vi "Begin.vi"(11 "Image Size":T1=enum."320x240") -> (0 "error out":errorcluster)   [LabVIEW 2012]
doc: "Called before other user functions, this VI is expected to open initial I/O refnums, load in file data, and do all program initialization. Notice that the <B>error out</B> terminal is simply used for data flow. Wiring it to other structures or subVIs ensures that this VI runs first."
uses:
  <vilib>/Rock Robotics/WPI/Camera/WPI_CameraImageSize.ctl
  <vilib>/Rock Robotics/WPI/DriverStation/WPI_DriverStationRobotMode2.ctl
  <vilib>/Rock Robotics/WPI/Joystick/WPI_JoystickDeviceEnum.ctl
  <vilib>/Rock Robotics/SystemInterfaces/DIO/FPGA_DIOPWMChannel.ctl
  <vilib>/Rock Robotics/SystemInterfaces/DIO/FPGA_DIORelayChannel.ctl
  <vilib>/Rock Robotics/SystemInterfaces/DIO/FPGA_DIOChannel.ctl
  <vilib>/Rock Robotics/SystemInterfaces/Typedef/FPGA_TypedefDigitalModule.ctl
  <vilib>/Rock Robotics/WPI/Solenoid/WPI_SolenoidChannel.ctl
  <vilib>/Rock Robotics/WPI/Encoder/WPI_EncoderType.ctl
  <vilib>/Rock Robotics/SystemInterfaces/Typedef/FPGA_TypedefAnalogModule.ctl
  <vilib>/Rock Robotics/SystemInterfaces/AI/FPGA_AIChannel.ctl
  RefnameEnum.ctl
  Sally_Dashboard_2014/DBNameEnum.ctl
  <vilib>/Rock Robotics/WPI/Solenoid/WPI_SolenoidValue.ctl
  <vilib>/Rock Robotics/WPI/SafetyOutput/WPI_SafetyOutputConfigMenu.ctl
  QueueInstruction.ctl
  SubsystemEnum.ctl
  ActionEnum.ctl
  TeleopData.ctl
  <vilib>/Rock Robotics/SystemInterfaces/CounterEncoderSourceConvertion/FPGA_CounterEncoderSourceConvertionLVSourceType.ctl
  <vilib>/Rock Robotics/SystemInterfaces/DIO/FPGA_DIODigitalSourceChannel.ctl
  <vilib>/Rock Robotics/SystemInterfaces/AnalogTrigger/FPGA_AnalogTriggerIndex.ctl
  <vilib>/Rock Robotics/SystemInterfaces/AnalogTrigger/FPGA_AnalogTriggerOutType.ctl
  Robot Global Data.vi
  <vilib>/Rock Robotics/WPI/RobotDrive/WPI_RobotDriveOpen2MotorWithTalon.vi
  <vilib>/Rock Robotics/WPI/MotorControl/WPI_MotorControlOpen Talon.vi
  <vilib>/Rock Robotics/WPI/Counter/WPI_CounterDigitalInputToDigitalSource.vi
  <vilib>/Rock Robotics/WPI/Solenoid/WPI_SolenoidOpenSingle.vi
  <vilib>/Rock Robotics/WPI/Solenoid/WPI_SolenoidSetEnum.vi
  <vilib>/Rock Robotics/WPI/MotorControl/WPI_MotorControlOpen Jaguar.vi
  <vilib>/Rock Robotics/WPI/Compressor/WPI_CompressorGetSetRefNum.vi
  <vilib>/Rock Robotics/WPI/Counter/WPI_CounterOpen UpDown Mode.vi
  <vilib>/Rock Robotics/WPI/Camera/WPI_CameraWhite Balance Values.ctl
  <vilib>/Rock Robotics/WPI/Camera/WPI_CameraExposure Values.ctl
  <vilib>/Rock Robotics/WPI/Camera/WPI_CameraFrameRate.ctl
  <vilib>/Rock Robotics/SystemInterfaces/AI/FPGA_AIGyroChannel.ctl
  <vilib>/Rock Robotics/SystemInterfaces/Typedef/FPGA_TypedefAnalogModuleForGyro.ctl
panel:
  in  "LowerLimit (v)":dbl=-1.0
  in  "UpperLimit (v)":dbl=1.0
  out "error out 2":errorcluster
  in  "Version String":string="TruongFramework 1.5.2"
  # "DON'T FORGET TO MAKE THIS DEFAULT"
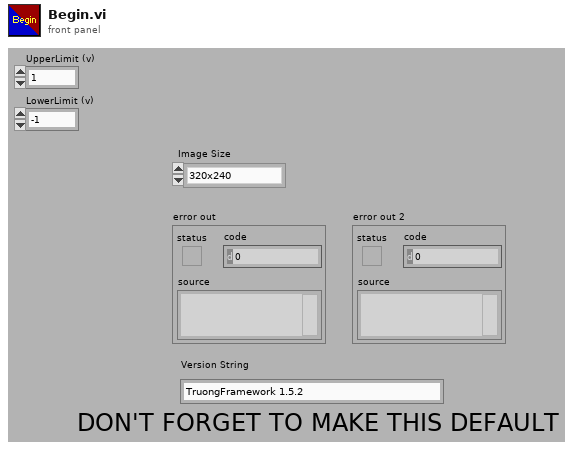
[diagram p1: front panel]
types:
  T1 = typedef "WPI_CameraImageSize.ctl" = enum16{"640x480", "320x240", "160x120"}
  T2 = typedef "TeleopData.ctl" = cluster{"cTankDriveLeft":dbl, "cTankDriveRight":dbl, "cHalfSpeed":bool, "cClimbWeight":bool, "cClimbStart":bool, "cRpmControl":dbl, "cAngleControl":dbl, "cQuickShoot":bool, "cLauncherWheel":bool, "cFirePneumatic":bool, "cPresetLow":bool, "cPresetHigh":bool, "cPresetClimbLow":bool, "cPresetClimbHigh":bool, "cLauncherAngle":bool, "cResetAngleEncoder":bool}
  T3 = typedef "QueueInstruction.ctl" = cluster{"Data":variant, "Subsystem":T4, "Action":T5}
  T4 = typedef "SubsystemEnum.ctl" = enum16{"TankDrive", "FirePneumatic", "Climber", "ClimbWeight", "ShooterAngle"}
  T5 = typedef "ActionEnum.ctl" = enum16{"Init", "SetValue"}
  T6 = typedef "WPI_SafetyOutputConfigMenu.ctl" = enum16{"Enable", "Disable"}
  T7 = typedef "WPI_SolenoidValue.ctl" = enum16{"Off", "On", "Forward", "Reverse"}
  T8 = typedef "RefnameEnum.ctl" = enum16{"FireLauncher", "Climber", "Shield", "TankDrive", "DriveEncoderL", "DriveEncoderR", "LauncherMotorRPM", "LauncherEncoderAnalog", "LauncherEncoderRPM", "ShooterLS", "DriveAlignLSLeft", "DriveAlignLSRight", "ClimbingLS", "LauncherEncoderAngle", "LauncherMotorAngle", "Gamepad1", "Gamepad2", "Compressor", "ClimbWeightSol3", "ClimbWeightSol4"}
  T9 = typedef "WPI_SolenoidChannel.ctl" = enum8{"Solenoid 1", "Solenoid 2", "Solenoid 3", "Solenoid 4", "Solenoid 5", "Solenoid 6", "Solenoid 7", "Solenoid 8", "Invalid"}
  T10 = typedef "FPGA_DIOChannel.ctl" = enum8{"DIO 1", "DIO 2", "DIO 3", "DIO 4", "DIO 5", "DIO 6", "DIO 7", "DIO 8", "DIO 9", "DIO 10", "DIO 11", "DIO 12", "DIO 13", "DIO 14", "Invalid"}
  T11 = typedef "FPGA_TypedefDigitalModule.ctl" = enum16{"Digital Module 1", "Digital Module 2"}
  T12 = typedef "DBNameEnum.ctl" = enum16{"AutoInstructions", "DriveLoopTime", "DriveAlignLSLeft", "DriveAlignLSRight", "Use2DriveAlign", "ClimbLS", "LauncherAngleMatches", "FrameworkVersion", "sLauncherAngle", "LauncherTargetAngle", "sLauncherRPM", "LauncherTargetRPM", "sDriveDistance", "LauncherMotorValue", "PullbackTol", "FireTol", "LauncherRPMTol", "LauncherAngleTol", "InitialWait", "WaitBetweenLaunch", "AnglePresets", "RPMPresets", "UseAngleEncoder", "UseLauncherEncoder", "UseLauncherPID", "QSWaitBeforeFire", "QSWaitBeforeRetract", "AngleForwardValue", "AngleBackwardValue", "UseClusterArray", "BackupAuto", "ReverseDriveIndicate", "HalfSpeedFactor"}
  T13 = typedef "FPGA_AIChannel.ctl" = enum8{"AI 1", "AI 2", "AI 3", "AI 4", "AI 5", "AI 6", "AI 7", "AI 8", "Invalid"}
  T14 = typedef "FPGA_TypedefAnalogModule.ctl" = enum16{"Analog Module 1", "Analog Module 2"}
  T15 = typedef "WPI_EncoderType.ctl" = enum16{"1x", "2x", "4x"}
  T16 = typedef "FPGA_DIORelayChannel.ctl" = enum8{"Relay 1", "Relay 2", "Relay 3", "Relay 4", "Relay 5", "Relay 6", "Relay 7", "Relay 8", "Invalid"}
  T17 = typedef "FPGA_DIOPWMChannel.ctl" = enum8{"PWM 1", "PWM 2", "PWM 3", "PWM 4", "PWM 5", "PWM 6", "PWM 7", "PWM 8", "PWM 9", "PWM 10", "Invalid"}
  T18 = typedef "WPI_JoystickDeviceEnum.ctl" = enum16{"USB 1", "USB 2", "USB 3", "USB 4", "Kinect 1", "Kinect 2"}
  T19 = typedef "WPI_DriverStationRobotMode2.ctl" = enum16{"Autonomous Disabled", "Autonomous Enabled", "Teleop Disabled", "Teleop Enabled", "Timeout", "Finish", "Test Disabled", "Test Enabled"}
  T20 = enum16{"Rising Edge", "Falling Edge", "Raising & Falling Edge", "Disabled"}
  T21 = typedef "WPI_DigitalInputDevRef.ctl" = cluster{"DevStatus":errorcluster, "DIO Channel":T10, "Digital Module":T11}
  T22 = typedef "FPGA_CounterEncoderSourceConvertionLVSourceType.ctl" = cluster{"DevStatus":errorcluster, "AnalogTriggerMode?":bool, "DigitalMode":cluster{"Digital Module":T11, "DIO Channel":T23}, "AnalogTriggerMode":cluster{"AnalogTriggerIndex":T24, "OutputType":T25}}
  T23 = typedef "FPGA_DIODigitalSourceChannel.ctl" = enum8{"DIO 1", "DIO 2", "DIO 3", "DIO 4", "DIO 5", "DIO 6", "DIO 7", "DIO 8", "DIO 9", "DIO 10", "DIO 11", "DIO 12", "DIO 13", "DIO 14", "Disabled"}
  T24 = typedef "FPGA_AnalogTriggerIndex.ctl" = enum8{"Trig 0", "Trig 1", "Trig 2", "Trig 3", "Trig 4", "Trig 5", "Trig 6", "Trig 7", "Invalid"}
  T25 = typedef "FPGA_AnalogTriggerOutType.ctl" = enum16{"InWindow", "TriggerState", "Rising", "Falling"}
  T26 = typedef "WPI_EncoderDevRef.ctl" = cluster{"DevStatus":errorcluster, "EncoderIndex":T27, "CounterIndex":T28, "DistancePerCount":dbl, "Decoding Type":T15}
  T27 = typedef "FPGA_EncoderIdx.ctl" = enum8{"Enc 0", "Enc 1", "Enc 2", "Enc 3", "Invalid"}
  T28 = typedef "FPGA_CounterCtrSystemIndex.ctl" = enum8{"Ctr 0", "Ctr 1", "Ctr 2", "Ctr 3", "Ctr 4", "Ctr 5", "Ctr 6", "Ctr 7", "Invalid"}
  T29 = typedef "WPI_CounterDevRef.ctl" = cluster{"DevStatus":errorcluster, "CntIndex":T28}
  T30 = typedef "FPGA_AIGyroChannel.ctl" = enum8{"AI 1", "AI 2", "Invalid"}
  T31 = typedef "FPGA_TypedefAnalogModuleForGyro.ctl" = enum16{"Analog Module 1"}
  T32 = typedef "WPI_GyroDevRef.ctl" = cluster{"DevStatus":errorcluster, "Analog Module":T14, "Analog Channel":T13, "Offset":dbl, "Gain (VoltsPerDegree/Second)":dbl}
  T33 = typedef "WPI_MotorControlDeviceRef.ctl" = cluster{"DeviceStatus":errorcluster, "Type":enum16{"PWM", "CAN"}, "PWM":cluster{"Digital Module":T11, "PWM Channel":T17, "DeadBand":T34}, "CAN":cluster{"Device Number":u8, "Control Mode":T35, "Semaphore":T36, "Max Vout":dbl}, "Invert":bool, "TransformRef":T37, "InvTransformRef":T37}
  T34 = typedef "WPI_PWMDeadband.ctl" = cluster{"Name":string, "maxPositivePwm":i32, "minPositivePwm":i32, "centerPwm":i32, "maxNegativePwm":i32, "minNegativePwm":i32, "angularRange":u16}
  T35 = typedef "WPI_CANJaguar_ControlMode.ctl" = enum8{"Percent VBus", "Current", "Speed", "Position", "Voltage"}
  T36 = typedef "Semaphore RefNum" = refnum<k1>
  T37 = typedef "WPI_PWMTransform_ConPane.ctl" = refnum<vi>
  T38 = typedef "WPI_RelayDevRef.ctl" = cluster{"DevStatus":errorcluster, "Relay Channel":T16, "Digital Module":T11, "Relay Direction":T39}
  T39 = typedef "WPI_RelayDirection.ctl" = enum16{"Both directions", "Forward only", "Reverse only"}
  T40 = typedef "WPI_SolenoidDevRef.ctl" = cluster{"DevStatus":errorcluster, "Solenoid Module":T41, "Forward Solenoid Channel":T9, "Reverse Solenoid Channel":T9}
  T41 = typedef "FPGA_TypedefSolenoidModule.ctl" = enum16{"Solenoid Module 1", "Solenoid Module 2"}
  T42 = typedef "WPI_CompressorDevRef.ctl" = cluster{"DevStatus":errorcluster, "DigitalInputDevRef":T21, "RelayDevRef":T38}
  T43 = typedef "WPI_RobotDriveDevRef.ctl" = cluster{"DevStatus":errorcluster, "Motors[]":T33[], "Square Inputs":bool, "Max Output":dbl, "Isochronous":bool}
  T44 = typedef "WPI_CameraFrameRate.ctl" = u32
  T45 = typedef "WPI_CameraExposure Values.ctl" = enum16{"Auto", "Flicker-free 50 Hz", "Flicker-free 60 Hz", "Hold current"}
  T46 = typedef "WPI_CameraWhite Balance Values.ctl" = enum16{"Auto", "Fixed indoor", "Fixed outdoor 1", "Fixed outdoor 2", "Fixed fluorescent 1", "Fixed fluorescent 2", "Hold current"}
  T47 = typedef "WPI_CameraDevRef.ctl" = cluster{"Camera Address":string, "CameraStatus":errorcluster, "Acquire Image Notifier":refnum<notifier>}
  T48 = typedef "WPI_JoystickDevRef.ctl" = cluster{"Device":T18}
  T49 = typedef "WPI_AnalogChannelDevRef.ctl" = cluster{"DevStatus":errorcluster, "Analog Module":T14, "Analog Channel":T13}
  T50 = typedef "FPGA_AnalogTriggerDevRef.ctl" = cluster{"DevStatus":errorcluster, "AnalogTriggerIndex":T24}
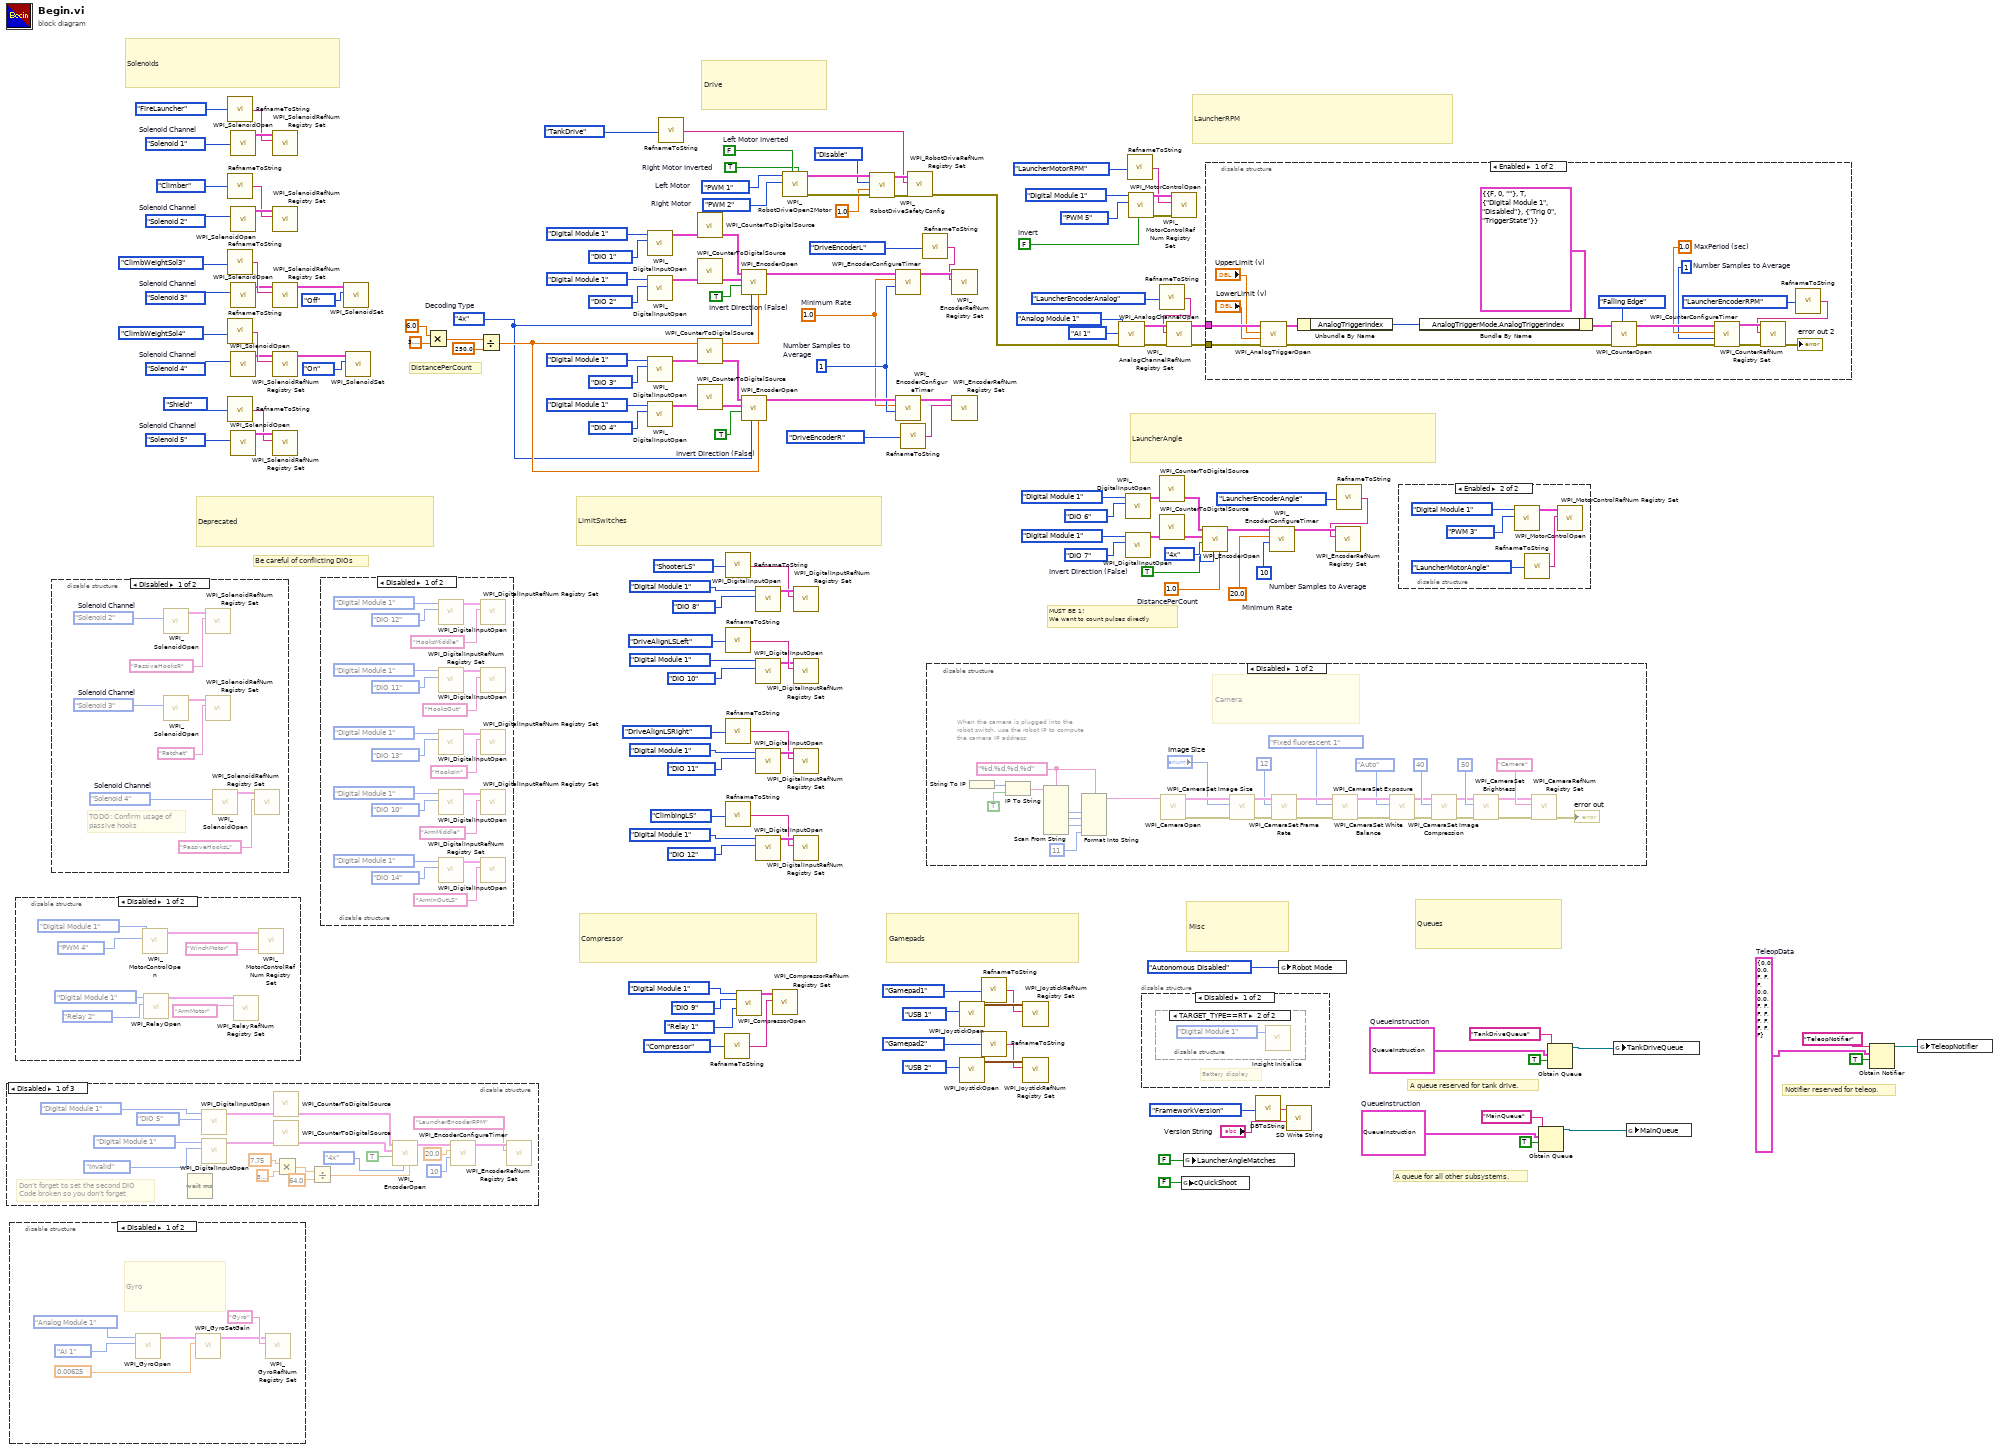
[diagram p0: block diagram]
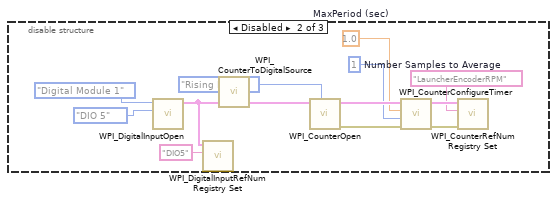
[diagram p8: hidden frame]
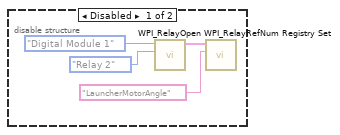
[diagram p12: hidden frame]
diagram:
  w4 = T2 {"cTankDriveLeft"=0.0, "cTankDriveRight"=0.0, "cHalfSpeed"=FALSE, "cClimbWeight"=FALSE, "cClimbStart"=FALSE, "cRpmControl"=0.0, "cAngleControl"=0.0, "cQuickShoot"=FALSE, "cLauncherWheel"=FALSE, "cFirePneumatic"=FALSE, "cPresetLow"=FALSE, "cPresetHigh"=FALSE, "cPresetClimbLow"=FALSE, "cPresetClimbHigh"=FALSE, "cLauncherAngle"=FALSE, "cResetAngleEncoder"=FALSE}  # TeleopData
  w9 = T3 {"Data"=variant, "Subsystem"=enum."TankDrive", "Action"=enum."Init"}  # QueueInstruction
  w10 = T3 {"Data"=variant, "Subsystem"=enum."TankDrive", "Action"=enum."Init"}  # QueueInstruction
  w24 = WPI_SolenoidChannel."Solenoid 4"  # Solenoid Channel
  w28 = WPI_SolenoidChannel."Solenoid 3"  # Solenoid Channel
  w84 = 1.0  # DistancePerCount
  w87 = TRUE  # Invert Direction (False)
  w88 = TRUE  # Invert Direction (False)
  w92 = WPI_SolenoidChannel."Solenoid 5"  # Solenoid Channel
  w94 = WPI_SolenoidChannel."Solenoid 2"  # Solenoid Channel
  w99 = TRUE  # Invert Direction (False)
  w101 = u8 10  # Number Samples to Average
  w102 = 20.0  # Minimum Rate
  w114 = WPI_SolenoidChannel."Solenoid 1"  # Solenoid Channel
  w89 = WPI_EncoderType."4x"  # Decoding Type
  w86 = u8 1  # Number Samples to Average
  w85 = 1.0  # Minimum Rate
  w143 = FALSE  # Invert
  w147 = FPGA_DIOPWMChannel."PWM 2"  # Right Motor
  w148 = FPGA_DIOPWMChannel."PWM 1"  # Left Motor
  w149 = TRUE  # Right Motor Inverted
  w150 = FALSE  # Left Motor Inverted
  # "Notifier reserved for teleop."
  # "A queue reserved for tank drive."
  # "A queue for all other subsystems."
  # "Queues"
  # "Be careful of conflicting DIOs"
  # "DistancePerCount"
  # "Deprecated"
  # "LimitSwitches"
  # "Compressor"
  # "Solenoids"
  # "LauncherAngle"
  # "LauncherRPM"
  # "Misc"
  # "Gamepads"
  # "Drive"
  # "MUST BE 1!\nWe want to count pulses directly"
  n1 = disable-structure shown="Disabled" {
    frame Disabled {
      # "Don't forget to set the second DIO\nCode broken so you don't forget"
      n2 = Wait (ms)() -> ()  [unwired: 1 in, 1 out]
      n3 = call <vilib>:"WPI_DigitalInputOpen.vi"("DIO Channel"=FPGA_DIOChannel."DIO 5", "Digital Module (Module 1)"=FPGA_TypedefDigitalModule."Digital Module 1") -> ("DigitalInputDevRef"=w173:T21)  [unwired: 1 in, 8 out]
      n4 = call <vilib>:"WPI_DigitalInputOpen.vi"("DIO Channel"=FPGA_DIOChannel."Invalid", "Digital Module (Module 1)"=FPGA_TypedefDigitalModule."Digital Module 1") -> ("DigitalInputDevRef"=w174:T21)  [unwired: 1 in, 8 out]
      n5 = call-poly <vilib>:"WPI_CounterToDigitalSource.vi"("DigitalInputDevRef"=w173) -> ("Digital Source"=w172:T22)  [unwired: 6 out]
      n6 = call-poly <vilib>:"WPI_CounterToDigitalSource.vi"("DigitalInputDevRef"=w174) -> ("Digital Source"=w175:T22)  [unwired: 6 out]
      n7 = Multiply(x=7.75, y=3.141592653589793) -> (x*y=w157:dbl)
      n8 = Divide(x=w157, y=64.0) -> (x/y=w160:dbl)
      n9 = call <vilib>:"WPI_EncoderOpen.vi"("DistancePerCount"=w160, "Decoding Type"=WPI_EncoderType."4x", "Invert Direction (False)"=TRUE, "BSource"=w175, "ASource"=w172) -> ("EncoderDevRef"=w169:T26)  [unwired: 3 in, 3 out]
      n10 = call <vilib>:"WPI_EncoderConfigureTimer.vi"("Number Samples to Average"=u8 10, "Minimum Rate"=20.0, "EncoderDevRef"=w169) -> ("EncoderDevRef"=w166:T26)  [unwired: 1 in, 7 out]
      n11 = call <vilib>:"WPI_EncoderRefNum Registry Set.vi"("refnum name"="LauncherEncoderRPM", "EncoderDevRef"=w166) -> ()  [unwired: 8 in, 2 out]
    }
    frame Disabled {
      w186 = u8 1  # Number Samples to Average
      w187 = 1.0  # MaxPeriod (sec)
      n12 = call <vilib>:"WPI_DigitalInputOpen.vi"("DIO Channel"=FPGA_DIOChannel."DIO 5", "Digital Module (Module 1)"=FPGA_TypedefDigitalModule."Digital Module 1") -> ("DigitalInputDevRef"=w177:T21)  [unwired: 8 in, 1 out]
      n13 = call <vilib>:"WPI_DigitalInputRefNum Registry Set.vi"("refnum name"="DIO5", "DigitalInputDevRef"=w177) -> ()  [unwired: 8 in, 2 out]
      n14 = call-poly <vilib>:"WPI_CounterToDigitalSource.vi"("DigitalInputDevRef"=w177) -> ("Digital Source"=w180:T22)  [unwired: 6 out]
      n15 = call-poly <vilib>:"WPI_CounterOpen.vi"("UpEdge"=T20."Rising Edge", "Up Source"=w180) -> ("error out"=w182:errorcluster, "CounterDevRef"=w188:T29)  [unwired: 8 in]
      n16 = call <vilib>:"WPI_CounterConfigureTimer.vi"("error in (no error)"=w182, "Number Samples to Average"=w186, "MaxPeriod (sec)"=w187, "CounterDevRef in"=w188) -> ("error out"=w181:errorcluster, "CounterDevRef out"=w185:T29)  [unwired: 6 in]
      n17 = call <vilib>:"WPI_CounterRefNum Registry Set.vi"("error in (no error)"=w181, "refnum name"="LauncherEncoderRPM", "CounterDevRef"=w185) -> ()  [unwired: 7 in, 2 out]
    }
    frame Enabled {
      # "LauncherRPM Deprecated"
    }
  }
  n18 = disable-structure shown="Disabled" {
    frame Disabled {
      # "Gyro"
      n19 = call <vilib>:"WPI_GyroOpen.vi"("Analog Channel"=FPGA_AIGyroChannel."AI 1", "Analog Module (Module 1)"=FPGA_TypedefAnalogModuleForGyro."Analog Module 1") -> ("GyroDevRef"=w191:T32)  [unwired: 7 in, 2 out]
      n20 = call <vilib>:"WPI_GyroSetGain.vi"("Gain (VoltsPerDegree/Second)"=0.00625, "GyroDevRef"=w191) -> ("GyroDevRef"=w190:T32)  [unwired: 8 in, 1 out]
      n21 = call <vilib>:"WPI_GyroRefNum Registry Set.vi"("refnum name"="Gyro", "GyroDevRef"=w190) -> ()  [unwired: 8 in, 2 out]
    }
    frame Enabled {
    }
  }
  n22 = disable-structure shown="Disabled" {
    frame Disabled {
      n23 = call-poly <vilib>:"WPI_MotorControlOpen.vi"("PWM Channel"=FPGA_DIOPWMChannel."PWM 4", "Digital Module (Module 1)"=FPGA_TypedefDigitalModule."Digital Module 1") -> ("MotorControlDeviceRef"=w200:T33)  [unwired: 8 in, 1 out]
      n24 = call <vilib>:"WPI_RelayOpen.vi"("Relay Channel"=FPGA_DIORelayChannel."Relay 2", "Digital Module (Module 1)"=FPGA_TypedefDigitalModule."Digital Module 1") -> ("RelayDevRef"=w196:T38)  [unwired: 8 in, 1 out]
      n25 = call <vilib>:"WPI_RelayRefNum Registry Set.vi"("refnum name"="ArmMotor", "RelayDevRef"=w196) -> ()  [unwired: 8 in, 2 out]
      n26 = call <vilib>:"WPI_MotorControlRefNum Registry Set.vi"("refnum name"="WinchMotor", "MotorControlDevRef"=w200) -> ()  [unwired: 8 in, 2 out]
    }
    frame Enabled {
    }
  }
  n27 = disable-structure shown="Disabled" {
    frame Disabled {
      w205 = WPI_SolenoidChannel."Solenoid 2"  # Solenoid Channel
      w208 = WPI_SolenoidChannel."Solenoid 4"  # Solenoid Channel
      w211 = WPI_SolenoidChannel."Solenoid 3"  # Solenoid Channel
      # "TODO: Confirm usage of\npassive hooks"
      n28 = call-poly <vilib>:"WPI_SolenoidOpen.vi"("Solenoid Channel"=w205) -> ("SolenoidDevRef"=w204:T40)  [unwired: 2 in, 8 out]
      n29 = call-poly <vilib>:"WPI_SolenoidOpen.vi"("Solenoid Channel"=w211) -> ("SolenoidDevRef"=w210:T40)  [unwired: 2 in, 8 out]
      n30 = call <vilib>:"WPI_SolenoidRefNum Registry Set.vi"("refnum name"="PassiveHooksR", "SolenoidDevRef"=w204) -> ()  [unwired: 8 in, 2 out]
      n31 = call <vilib>:"WPI_SolenoidRefNum Registry Set.vi"("refnum name"="Ratchet", "SolenoidDevRef"=w210) -> ()  [unwired: 8 in, 2 out]
      n32 = call-poly <vilib>:"WPI_SolenoidOpen.vi"("Solenoid Channel"=w208) -> ("SolenoidDevRef"=w207:T40)  [unwired: 2 in, 8 out]
      n33 = call <vilib>:"WPI_SolenoidRefNum Registry Set.vi"("refnum name"="PassiveHooksL", "SolenoidDevRef"=w207) -> ()  [unwired: 8 in, 2 out]
    }
    frame Enabled {
    }
  }
  n34 = call "RefnameToString.vi"("Enum"=RefnameEnum."FireLauncher") -> ("Refname"=w67:string)
  n35 = call "RefnameToString.vi"("Enum"=RefnameEnum."Climber") -> ("Refname"=w65:string)
  n36 = call "RefnameToString.vi"("Enum"=RefnameEnum."ClimbWeightSol3") -> ("Refname"=w31:string)
  n37 = call "RefnameToString.vi"("Enum"=RefnameEnum."ClimbWeightSol4") -> ("Refname"=w27:string)
  n38 = call "RefnameToString.vi"("Enum"=RefnameEnum."Shield") -> ("Refname"=w63:string)
  n39 = call-poly <vilib>:"WPI_SolenoidOpen.vi"("Solenoid Channel"=w114) -> ("SolenoidDevRef"=w113:T40)  [unwired: 2 in, 8 out]
  n40 = call-poly <vilib>:"WPI_SolenoidOpen.vi"("Solenoid Channel"=w94) -> ("SolenoidDevRef"=w93:T40)  [unwired: 2 in, 8 out]
  n41 = call-poly <vilib>:"WPI_SolenoidOpen.vi"("Solenoid Channel"=w28) -> ("SolenoidDevRef"=w29:T40)  [unwired: 2 in, 8 out]
  n42 = call-poly <vilib>:"WPI_SolenoidOpen.vi"("Solenoid Channel"=w24) -> ("SolenoidDevRef"=w25:T40)  [unwired: 2 in, 8 out]
  n43 = call-poly <vilib>:"WPI_SolenoidOpen.vi"("Solenoid Channel"=w92) -> ("SolenoidDevRef"=w91:T40)  [unwired: 2 in, 8 out]
  n44 = call <vilib>:"WPI_SolenoidRefNum Registry Set.vi"("refnum name"=w67, "SolenoidDevRef"=w113) -> ()  [unwired: 8 in, 2 out]
  n45 = call <vilib>:"WPI_SolenoidRefNum Registry Set.vi"("refnum name"=w65, "SolenoidDevRef"=w93) -> ()  [unwired: 8 in, 2 out]
  n46 = call <vilib>:"WPI_SolenoidRefNum Registry Set.vi"("refnum name"=w31, "SolenoidDevRef"=w29) -> ("SolenoidDevRef"=w23:T40)  [unwired: 8 in, 1 out]
  n47 = call <vilib>:"WPI_SolenoidRefNum Registry Set.vi"("refnum name"=w27, "SolenoidDevRef"=w25) -> ("SolenoidDevRef"=w22:T40)  [unwired: 8 in, 1 out]
  n48 = call <vilib>:"WPI_SolenoidRefNum Registry Set.vi"("refnum name"=w63, "SolenoidDevRef"=w91) -> ()  [unwired: 8 in, 2 out]
  n49 = disable-structure shown="Disabled" {
    frame Disabled {
      n50 = call <vilib>:"WPI_DigitalInputOpen.vi"("DIO Channel"=FPGA_DIOChannel."DIO 12", "Digital Module (Module 1)"=FPGA_TypedefDigitalModule."Digital Module 1") -> ("DigitalInputDevRef"=w215:T21)  [unwired: 8 in, 1 out]
      n51 = call <vilib>:"WPI_DigitalInputOpen.vi"("DIO Channel"=FPGA_DIOChannel."DIO 11", "Digital Module (Module 1)"=FPGA_TypedefDigitalModule."Digital Module 1") -> ("DigitalInputDevRef"=w219:T21)  [unwired: 8 in, 1 out]
      n52 = call <vilib>:"WPI_DigitalInputOpen.vi"("DIO Channel"=FPGA_DIOChannel."DIO 13", "Digital Module (Module 1)"=FPGA_TypedefDigitalModule."Digital Module 1") -> ("DigitalInputDevRef"=w223:T21)  [unwired: 8 in, 1 out]
      n53 = call <vilib>:"WPI_DigitalInputOpen.vi"("DIO Channel"=FPGA_DIOChannel."DIO 10", "Digital Module (Module 1)"=FPGA_TypedefDigitalModule."Digital Module 1") -> ("DigitalInputDevRef"=w227:T21)  [unwired: 8 in, 1 out]
      n54 = call <vilib>:"WPI_DigitalInputOpen.vi"("DIO Channel"=FPGA_DIOChannel."DIO 14", "Digital Module (Module 1)"=FPGA_TypedefDigitalModule."Digital Module 1") -> ("DigitalInputDevRef"=w231:T21)  [unwired: 8 in, 1 out]
      n55 = call <vilib>:"WPI_DigitalInputRefNum Registry Set.vi"("refnum name"="HooksMiddle", "DigitalInputDevRef"=w215) -> ()  [unwired: 8 in, 2 out]
      n56 = call <vilib>:"WPI_DigitalInputRefNum Registry Set.vi"("refnum name"="HooksOut", "DigitalInputDevRef"=w219) -> ()  [unwired: 8 in, 2 out]
      n57 = call <vilib>:"WPI_DigitalInputRefNum Registry Set.vi"("refnum name"="HooksIn", "DigitalInputDevRef"=w223) -> ()  [unwired: 8 in, 2 out]
      n58 = call <vilib>:"WPI_DigitalInputRefNum Registry Set.vi"("refnum name"="ArmMiddle", "DigitalInputDevRef"=w227) -> ()  [unwired: 8 in, 2 out]
      n59 = call <vilib>:"WPI_DigitalInputRefNum Registry Set.vi"("refnum name"="ArmInOutLS", "DigitalInputDevRef"=w231) -> ()  [unwired: 8 in, 2 out]
    }
    frame Enabled {
    }
  }
  n60 = call-poly <vilib>:"WPI_SolenoidSet.vi"("Value"=WPI_SolenoidValue."Off", "SolenoidDevRef"=w23) -> ()  [unwired: 8 in, 2 out]
  n61 = call-poly <vilib>:"WPI_SolenoidSet.vi"("Value"=WPI_SolenoidValue."On", "SolenoidDevRef"=w22) -> ()  [unwired: 8 in, 2 out]
  n62 = Multiply(x=6.0, y=3.141592653589793) -> (x*y=w96:dbl)
  n63 = Divide(x=w96, y=250.0) -> (x/y=w90:dbl)
  n64 = call <vilib>:"WPI_DigitalInputOpen.vi"("DIO Channel"=FPGA_DIOChannel."DIO 1", "Digital Module (Module 1)"=FPGA_TypedefDigitalModule."Digital Module 1") -> ("DigitalInputDevRef"=w135:T21)  [unwired: 1 in, 8 out]
  n65 = call <vilib>:"WPI_DigitalInputOpen.vi"("DIO Channel"=FPGA_DIOChannel."DIO 2", "Digital Module (Module 1)"=FPGA_TypedefDigitalModule."Digital Module 1") -> ("DigitalInputDevRef"=w136:T21)  [unwired: 1 in, 8 out]
  n66 = call <vilib>:"WPI_DigitalInputOpen.vi"("DIO Channel"=FPGA_DIOChannel."DIO 3", "Digital Module (Module 1)"=FPGA_TypedefDigitalModule."Digital Module 1") -> ("DigitalInputDevRef"=w122:T21)  [unwired: 1 in, 8 out]
  n67 = call <vilib>:"WPI_DigitalInputOpen.vi"("DIO Channel"=FPGA_DIOChannel."DIO 4", "Digital Module (Module 1)"=FPGA_TypedefDigitalModule."Digital Module 1") -> ("DigitalInputDevRef"=w123:T21)  [unwired: 1 in, 8 out]
  n68 = call "RefnameToString.vi"("Enum"=RefnameEnum."TankDrive") -> ("Refname"=w15:string)
  n69 = call-poly <vilib>:"WPI_CounterToDigitalSource.vi"("DigitalInputDevRef"=w135) -> ("Digital Source"=w134:T22)  [unwired: 6 out]
  n70 = call-poly <vilib>:"WPI_CounterToDigitalSource.vi"("DigitalInputDevRef"=w136) -> ("Digital Source"=w137:T22)  [unwired: 6 out]
  n71 = call-poly <vilib>:"WPI_CounterToDigitalSource.vi"("DigitalInputDevRef"=w122) -> ("Digital Source"=w121:T22)  [unwired: 6 out]
  n72 = call-poly <vilib>:"WPI_CounterToDigitalSource.vi"("DigitalInputDevRef"=w123) -> ("Digital Source"=w124:T22)  [unwired: 6 out]
  n73 = call "RefnameToString.vi"("Enum"=RefnameEnum."Compressor") -> ("Refname"=w44:string)
  n74 = call "RefnameToString.vi"("Enum"=RefnameEnum."ShooterLS") -> ("Refname"=w50:string)
  n75 = call "RefnameToString.vi"("Enum"=RefnameEnum."DriveAlignLSLeft") -> ("Refname"=w37:string)
  n76 = call "RefnameToString.vi"("Enum"=RefnameEnum."DriveAlignLSRight") -> ("Refname"=w48:string)
  n77 = call "RefnameToString.vi"("Enum"=RefnameEnum."ClimbingLS") -> ("Refname"=w46:string)
  n78 = call <vilib>:"WPI_CompressorOpen.vi"("Pressure Switch Digital Module (Module 1)"=FPGA_TypedefDigitalModule."Digital Module 1" ("Pressure Switch\nand Relay Module"), "Pressure Switch DIO Channel"=FPGA_DIOChannel."DIO 9" ("Pressure Switch Channel"), "Relay Channel"=FPGA_DIORelayChannel."Relay 1") -> ("CompressorDevRef"=w138:T42)  [unwired: 2 in, 10 out]
  n79 = call <vilib>:"WPI_EncoderOpen.vi"("DistancePerCount"=w90, "Decoding Type"=w89, "Invert Direction (False)"=w88, "BSource"=w137, "ASource"=w134) -> ("EncoderDevRef"=w131:T26)  [unwired: 3 in, 3 out]
  n80 = call <vilib>:"WPI_EncoderOpen.vi"("DistancePerCount"=w90, "Decoding Type"=w89, "Invert Direction (False)"=w87, "BSource"=w124, "ASource"=w121) -> ("EncoderDevRef"=w118:T26)  [unwired: 3 in, 3 out]
  n81 = call <vilib>:"WPI_DigitalInputOpen.vi"("DIO Channel"=FPGA_DIOChannel."DIO 8", "Digital Module (Module 1)"=FPGA_TypedefDigitalModule."Digital Module 1") -> ("DigitalInputDevRef"=w127:T21)  [unwired: 8 in, 1 out]
  n82 = call <vilib>:"WPI_DigitalInputOpen.vi"("DIO Channel"=FPGA_DIOChannel."DIO 10", "Digital Module (Module 1)"=FPGA_TypedefDigitalModule."Digital Module 1") -> ("DigitalInputDevRef"=w33:T21)  [unwired: 8 in, 1 out]
  n83 = call <vilib>:"WPI_DigitalInputOpen.vi"("DIO Channel"=FPGA_DIOChannel."DIO 11", "Digital Module (Module 1)"=FPGA_TypedefDigitalModule."Digital Module 1") -> ("DigitalInputDevRef"=w77:T21)  [unwired: 8 in, 1 out]
  n84 = call <vilib>:"WPI_DigitalInputOpen.vi"("DIO Channel"=FPGA_DIOChannel."DIO 12", "Digital Module (Module 1)"=FPGA_TypedefDigitalModule."Digital Module 1") -> ("DigitalInputDevRef"=w71:T21)  [unwired: 8 in, 1 out]
  n85 = call <vilib>:"WPI_CompressorRefNum Registry Set.vi"("refnum name"=w44, "CompressorDevRef"=w138) -> ()  [unwired: 8 in, 2 out]
  n86 = call-poly <vilib>:"WPI_RobotDriveOpen2Motor.vi"("Right Motor Inverted"=w149, "Left Motor Inverted"=w150, "Right Motor"=w147, "Left Motor"=w148) -> ("error out"=w16:errorcluster, "RobotDriveDevRef"=w19:T43)  [unwired: 6 in]
  n87 = call <vilib>:"WPI_DigitalInputRefNum Registry Set.vi"("refnum name"=w50, "DigitalInputDevRef"=w127) -> ()  [unwired: 8 in, 2 out]
  n88 = call <vilib>:"WPI_DigitalInputRefNum Registry Set.vi"("refnum name"=w37, "DigitalInputDevRef"=w33) -> ()  [unwired: 8 in, 2 out]
  n89 = call <vilib>:"WPI_DigitalInputRefNum Registry Set.vi"("refnum name"=w48, "DigitalInputDevRef"=w77) -> ()  [unwired: 8 in, 2 out]
  n90 = call <vilib>:"WPI_DigitalInputRefNum Registry Set.vi"("refnum name"=w46, "DigitalInputDevRef"=w71) -> ()  [unwired: 8 in, 2 out]
  n91 = call <vilib>:"WPI_RobotDriveSafetyConfig.vi"("error in (no error)"=w16, "timeout (s)"=1.0, "mode"=WPI_SafetyOutputConfigMenu."Disable", "RobotDriveDevRef"=w19) -> ("error out"=w17:errorcluster, "RobotDriveDevRef"=w18:T43)  [unwired: 6 in]
  n92 = call <vilib>:"WPI_EncoderConfigureTimer.vi"("Number Samples to Average"=w86, "Minimum Rate"=w85, "EncoderDevRef"=w131) -> ("EncoderDevRef"=w128:T26)  [unwired: 1 in, 7 out]
  n93 = call <vilib>:"WPI_EncoderConfigureTimer.vi"("Number Samples to Average"=w86, "Minimum Rate"=w85, "EncoderDevRef"=w118) -> ("EncoderDevRef"=w115:T26)  [unwired: 1 in, 7 out]
  n94 = call "RefnameToString.vi"("Enum"=RefnameEnum."DriveEncoderR") -> ("Refname"=w58:string)
  n95 = call <vilib>:"WPI_RobotDriveRefNum Registry Set.vi"("error in (no error)"=w17, "refnum name"=w15, "RobotDriveDevRef"=w18) -> ("error out"=w74:errorcluster)  [unwired: 7 in, 1 out]
  n96 = call "RefnameToString.vi"("Enum"=RefnameEnum."DriveEncoderL") -> ("Refname"=w60:string)
  n97 = disable-structure shown="Disabled" {
    frame Disabled {
      w234 = "%d.%d.%d.%d" ("format string")
      # "Camera"
      # "When the camera is plugged into the\nrobot switch, use the robot IP to compute\nthe camera IP address"
      n98 = String To IP() -> (0:w241:u32)  [unwired: 1 in]
      n99 = IP To String(1:TRUE ("dot notation? (F)"), 2:w241) -> (0:w239:string)
      n100 = Scan From String(format string=w234, input string=w239) -> (output 1=w238:i32, output 2=w237:i32, output 3=w236:i32)  [unwired: 7 in, 3 out]
      n101 = Format Into String(format string=w234, w238, w237, w236, 11 ("Compression")) -> (resulting string=w233:string)  [unwired: 2 in, 1 out]
      n102 = call <vilib>:"WPI_CameraOpen.vi"("Camera Address"=w233) -> ("error out"=w253:errorcluster, "CameraDevRef"=w254:T47)  [unwired: 1 in, 8 out]
      n103 = call <vilib>:"WPI_CameraSet Image Size.vi"("error in (no error)"=w253, "Image Size"="Image Size", "CameraDevRef"=w254) -> ("error out"=w252:errorcluster, "CameraDevRef Out"=w255:T47)  [unwired: 7 out]
      n104 = call <vilib>:"WPI_CameraSet Frame Rate.vi"("error in (no error)"=w252, "Frame Rate (fps)"=T44 12, "CameraDevRef"=w255) -> ("error out"=w251:errorcluster, "CameraDevRef Out"=w257:T47)  [unwired: 7 out]
      n105 = call <vilib>:"WPI_CameraSet White Balance.vi"("error in (no error)"=w251, "White Balance"=WPI_CameraWhite_Balance_Values."Fixed fluorescent 1", "CameraDevRef"=w257) -> ("error out"=w250:errorcluster, "CameraDevRef Out"=w256:T47)  [unwired: 7 out]
      n106 = call <vilib>:"WPI_CameraSet Exposure.vi"("error in (no error)"=w250, "Exposure"=WPI_CameraExposure_Values."Auto", "CameraDevRef"=w256) -> ("error out"=w249:errorcluster, "CameraDevRef Out"=w259:T47)  [unwired: 7 out]
      n107 = call <vilib>:"WPI_CameraSet Image Compression.vi"("error in (no error)"=w249, "Compression"=40, "CameraDevRef"=w259) -> ("error out"=w248:errorcluster, "CameraDevRef Out"=w258:T47)  [unwired: 7 out]
      n108 = call <vilib>:"WPI_CameraSet Brightness.vi"("error in (no error)"=w248, "Brightness"=50, "CameraDevRef"=w258) -> ("error out"=w246:errorcluster, "CameraDevRef Out"=w247:T47)  [unwired: 7 out]
      n109 = call <vilib>:"WPI_CameraRefNum Registry Set.vi"("error in (no error)"=w246, "refnum name"="Camera", "CameraDevRef"=w247) -> ("error out"=→"error out":errorcluster)  [unwired: 8 out]
    }
    frame Enabled {
    }
  }
  n110 = call <vilib>:"WPI_EncoderRefNum Registry Set.vi"("refnum name"=w60, "EncoderDevRef"=w128) -> ()  [unwired: 8 in, 2 out]
  n111 = call <vilib>:"WPI_EncoderRefNum Registry Set.vi"("refnum name"=w58, "EncoderDevRef"=w115) -> ()  [unwired: 8 in, 2 out]
  n112 = call <vilib>:"WPI_JoystickOpen.vi"("JoystickDevice"=WPI_JoystickDeviceEnum."USB 1") -> ("JoystickDevRef"=w154:T48)  [unwired: 10 in]
  n113 = call <vilib>:"WPI_JoystickOpen.vi"("JoystickDevice"=WPI_JoystickDeviceEnum."USB 2") -> ("JoystickDevRef"=w151:T48)  [unwired: 10 in]
  n114 = call "RefnameToString.vi"("Enum"=RefnameEnum."Gamepad1") -> ("Refname"=w40:string)
  n115 = call "RefnameToString.vi"("Enum"=RefnameEnum."Gamepad2") -> ("Refname"=w42:string)
  n116 = call <vilib>:"WPI_JoystickRefNum Registry Set.vi"("refnum name"=w40, "JoystickDevRef"=w154) -> ()  [unwired: 8 in, 2 out]
  n117 = call <vilib>:"WPI_JoystickRefNum Registry Set.vi"("refnum name"=w42, "JoystickDevRef"=w151) -> ()  [unwired: 8 in, 2 out]
  n118 = call <vilib>:"WPI_AnalogChannelOpen.vi"("error in (no error)"=w74, "Analog Channel"=FPGA_AIChannel."AI 1", "Analog Module (Module 1)"=FPGA_TypedefAnalogModule."Analog Module 1") -> ("error out"=w79:errorcluster, "AIDeviceRef"=w78:T49)  [unwired: 7 in]
  n119 = call <vilib>:"WPI_DigitalInputOpen.vi"("DIO Channel"=FPGA_DIOChannel."DIO 6", "Digital Module (Module 1)"=FPGA_TypedefDigitalModule."Digital Module 1") -> ("DigitalInputDevRef"=w110:T21)  [unwired: 1 in, 8 out]
  n120 = call <vilib>:"WPI_DigitalInputOpen.vi"("DIO Channel"=FPGA_DIOChannel."DIO 7", "Digital Module (Module 1)"=FPGA_TypedefDigitalModule."Digital Module 1") -> ("DigitalInputDevRef"=w111:T21)  [unwired: 1 in, 8 out]
  n121 = call "RefnameToString.vi"("Enum"=RefnameEnum."LauncherMotorRPM") -> ("Refname"=w56:string)
  n122 = call-poly <vilib>:"WPI_MotorControlOpen.vi"("Invert"=w143, "PWM Channel"=FPGA_DIOPWMChannel."PWM 5", "Digital Module (Module 1)"=FPGA_TypedefDigitalModule."Digital Module 1") -> ("error out"=w142:errorcluster, "MotorControlDeviceRef"=w146:T33)  [unwired: 7 in]
  n123 = disable-structure shown="Disabled" {
    frame Disabled {
      # "Battery display"
      n124 = disable-structure shown="TARGET_TYPE==RT" {
        frame condition #0 {
        }
        frame condition #1 (active) {
          n125 = call "Insight Initialize.vi"("Digital Module"=FPGA_TypedefDigitalModule."Digital Module 1") -> ()  [unwired: 2 in]
        }
      }
    }
    frame Enabled {
    }
  }
  n126 = call "RefnameToString.vi"("Enum"=RefnameEnum."LauncherEncoderAnalog") -> ("Refname"=w54:string)
  n127 = call-poly <vilib>:"WPI_CounterToDigitalSource.vi"("DigitalInputDevRef"=w110) -> ("Digital Source"=w109:T22)  [unwired: 6 out]
  n128 = call-poly <vilib>:"WPI_CounterToDigitalSource.vi"("DigitalInputDevRef"=w111) -> ("Digital Source"=w112:T22)  [unwired: 6 out]
  n129 = call <vilib>:"WPI_AnalogChannelRefNum Registry Set.vi"("error in (no error)"=w79, "refnum name"=w54, "AIDeviceRef"=w78) -> ("error out"=w72:errorcluster, "AIDeviceRef"=w73:T49)  [unwired: 7 in]
  n130 = call <vilib>:"WPI_MotorControlRefNum Registry Set.vi"("error in (no error)"=w142, "refnum name"=w56, "MotorControlDevRef"=w146) -> ()  [unwired: 7 in, 2 out]
  n131 = global write "Robot Global Data.vi" "cQuickShoot"(FALSE) -> ()
  n132 = global write "Robot Global Data.vi" "LauncherAngleMatches"(FALSE) -> ()
  n133 = call <vilib>:"WPI_EncoderOpen.vi"("DistancePerCount"=w84, "Decoding Type"=WPI_EncoderType."4x", "Invert Direction (False)"=w99, "BSource"=w112, "ASource"=w109) -> ("EncoderDevRef"=w106:T26)  [unwired: 3 in, 3 out]
  n134 = disable-structure shown="Enabled" {
    disable-tunnel: w73 -> [w269 _]
    disable-tunnel: w72 -> [w268 _]
    frame Enabled {
      w278 = u8 1  # Number Samples to Average
      w279 = 1.0  # MaxPeriod (sec)
      n135 = call <vilib>:"WPI_AnalogTriggerOpen.vi"("error in (no error)"=w268, "LowerLimit (v)"="LowerLimit (v)", "UpperLimit (v)"="UpperLimit (v)", "AnalogTriggerSource"=w269) -> ("error out"=w282:errorcluster, "AnalogTriggerDevRef"=w277:T50)  [unwired: 6 in]
      n136 = Unbundle By Name(w277) -> ("AnalogTriggerIndex"=w276:T24)
      n137 = Bundle By Name(cluster=T22 {"DevStatus"={"status"=FALSE, "code"=0, "source"=""}, "AnalogTriggerMode?"=TRUE, "DigitalMode"={"Digital Module"=enum."Digital Module 1", "DIO Channel"=enum."Disabled"}, "AnalogTriggerMode"={"AnalogTriggerIndex"=enum."Trig 0", "OutputType"=enum."TriggerState"}} ("Source"), "AnalogTriggerMode.AnalogTriggerIndex"=w276) -> (w274:T22)
      n138 = call-poly <vilib>:"WPI_CounterOpen.vi"("UpEdge"=T20."Falling Edge" ("UpEdge 1"), "error in (no error)"=w282, "Up Source"=w274) -> ("error out"=w280:errorcluster, "CounterDevRef"=w281:T29)  [unwired: 7 in]
      n139 = call <vilib>:"WPI_CounterConfigureTimer.vi"("error in (no error)"=w280, "Number Samples to Average"=w278, "MaxPeriod (sec)"=w279, "CounterDevRef in"=w281) -> ("error out"=w271:errorcluster, "CounterDevRef out"=w272:T29)  [unwired: 6 in]
      n140 = call "RefnameToString.vi"("Enum"=RefnameEnum."LauncherEncoderRPM") -> ("Refname"=w266:string)
      n141 = call <vilib>:"WPI_CounterRefNum Registry Set.vi"("error in (no error)"=w271, "refnum name"=w266, "CounterDevRef"=w272) -> ("error out"=→"error out 2":errorcluster)  [unwired: 7 in, 1 out]
    }
    frame Disabled {
    }
  }
  n142 = call "DBToString.vi"("Enum"=DBNameEnum."FrameworkVersion") -> ("Refname"=w38:string)
  n143 = call <vilib>:"WPI_EncoderConfigureTimer.vi"("Number Samples to Average"=w101, "Minimum Rate"=w102, "EncoderDevRef"=w106) -> ("EncoderDevRef"=w103:T26)  [unwired: 1 in, 7 out]
  n144 = global write "Robot Global Data.vi" "Robot Mode"(WPI_DriverStationRobotMode2."Autonomous Disabled" ("Robot Mode")) -> ()
  n145 = call <vilib>:"SD Write String.vi"("String"="Version String", "Name"=w38) -> ()  [unwired: 8 in, 2 out]
  n146 = call "RefnameToString.vi"("Enum"=RefnameEnum."LauncherEncoderAngle") -> ("Refname"=w52:string)
  n147 = call <vilib>:"WPI_EncoderRefNum Registry Set.vi"("refnum name"=w52, "EncoderDevRef"=w103) -> ()  [unwired: 8 in, 2 out]
  n148 = disable-structure shown="Enabled" {
    frame Disabled {
      n149 = call <vilib>:"WPI_RelayOpen.vi"("Relay Channel"=FPGA_DIORelayChannel."Relay 2", "Digital Module (Module 1)"=FPGA_TypedefDigitalModule."Digital Module 1") -> ("RelayDevRef"=w284:T38)  [unwired: 8 in, 1 out]
      n150 = call <vilib>:"WPI_RelayRefNum Registry Set.vi"("refnum name"="LauncherMotorAngle", "RelayDevRef"=w284) -> ()  [unwired: 8 in, 2 out]
    }
    frame Enabled {
      n151 = call-poly <vilib>:"WPI_MotorControlOpen.vi"("PWM Channel"=FPGA_DIOPWMChannel."PWM 3", "Digital Module (Module 1)"=FPGA_TypedefDigitalModule."Digital Module 1") -> ("MotorControlDeviceRef"=w290:T33)  [unwired: 8 in, 1 out]
      n152 = call "RefnameToString.vi"("Enum"=RefnameEnum."LauncherMotorAngle") -> ("Refname"=w287:string)
      n153 = call <vilib>:"WPI_MotorControlRefNum Registry Set.vi"("refnum name"=w287, "MotorControlDevRef"=w290) -> ()  [unwired: 8 in, 2 out]
    }
  }
  n154 = Obtain Queue(name (unnamed)="MainQueue", element data type=w9, create if not found? (T)=TRUE) -> (queue out=w2:refnum<queue>)  [unwired: 2 in, 2 out]
  n155 = Obtain Queue(name (unnamed)="TankDriveQueue", element data type=w10, create if not found? (T)=TRUE) -> (queue out=w3:refnum<queue>)  [unwired: 2 in, 2 out]
  n156 = global write "Robot Global Data.vi" "TankDriveQueue"(w3) -> ()
  n157 = global write "Robot Global Data.vi" "MainQueue"(w2) -> ()
  n158 = Obtain Notifier(name (unnamed)="TeleopNotifier", notification data type=w4, create if not found? (T)=TRUE) -> (notifier out=w1:refnum<notifier>)  [unwired: 1 in, 2 out]
  n159 = global write "Robot Global Data.vi" "TeleopNotifier"(w1) -> ()
